vi "manage loss communication.vi"(8 "error in (no error)":errorcluster, 11 "Channel in":refnum<class "Channel.lvclass">) -> (0 "error out":errorcluster, 3 "Channel out":refnum<class "Channel.lvclass">)   [LabVIEW 2018, in "Channel.lvclass"]
uses:
  Channel.lvclass
  Server/Server.lvclass
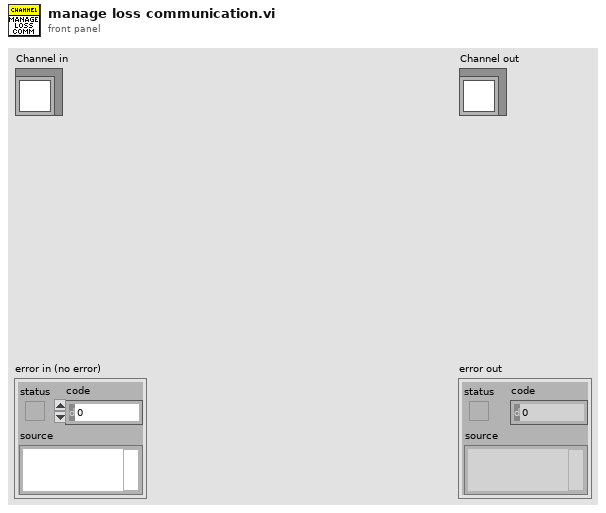
[diagram p1: front panel]
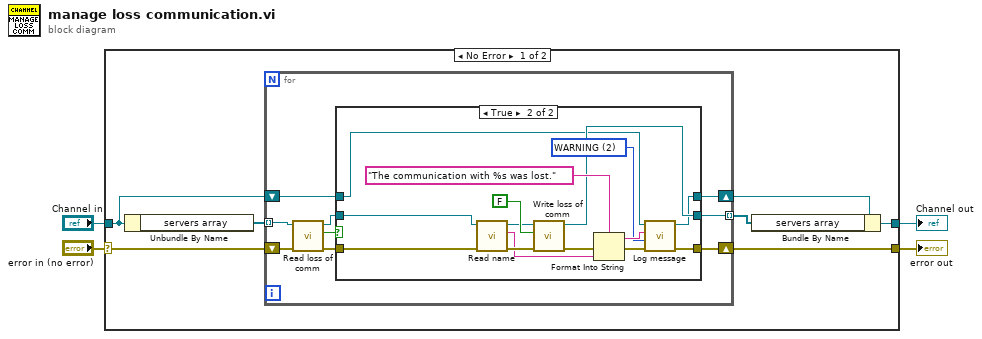
[diagram p0: block diagram]
diagram:
  n1 = case shown="No Error" "error in (no error)" {
    selector: "error in (no error)" -> [w10 w40]
    tunnel: [w9 w40] -> w3
    tunnel: [w7 w39] -> w1
    tunnel: "Channel in" -> [w11 w39]
    frame No Error {
      n2 = Unbundle By Name(w11) -> ("servers array"=w6:refnum<class "Server.lvclass">[])
      n3 = for {
        shift-right: [w19] -> w8
        shift-left: w11 -> [w20]
        shift-right: [w18] -> w9
        shift-left: w10 -> [w15]
        tunnel: w6 -> [w16] mode=indexing
        tunnel: [w12] -> w5 mode=indexing
        n4 = call-dynamic "Read loss of comm.vi"("error in (no error)"=w15, "Server in"=w16) -> ("error out"=w14:errorcluster, "loss of comm"=w13:bool, "Server out"=w17:refnum<class "Server.lvclass">)  [unwired: 7 in]
        n5 = case shown="True" w13 {
          tunnel: w20 -> [w23 w26]
          tunnel: [w23 w25] -> w19
          tunnel: [w22 w27] -> w18
          tunnel: w17 -> [w21 w34]
          tunnel: w14 -> [w22 w33]
          tunnel: [w21 w35] -> w12
          frame False {
          }
          frame True {
            w24 = u16 2 items=[" DEBBUG ", "  INFO  ", "WARNING ", " ERROR  ", "CRITICAL"] ("log level")
            n6 = call-dynamic "Read name.vi"("error in (no error)"=w33, "Server in"=w34) -> ("error out"=w32:errorcluster, "name"=w30:string, "Server out"=w31:refnum<class "Server.lvclass">)  [unwired: 7 in]
            n7 = call-dynamic "Write loss of comm.vi"("error in (no error)"=w32, "loss of comm"=FALSE, "Server in"=w31) -> ("error out"=w37:errorcluster, "Server out"=w35:refnum<class "Server.lvclass">)  [unwired: 7 in]
            n8 = Format Into String(format string="The communication with %s was lost.", error in=w37, w30) -> (resulting string=w29:string, error out=w28:errorcluster)  [unwired: 1 in]
            n9 = call "Log message.vi"("error in (no error)"=w28, "log level"=w24, "String"=w29, "Channel in"=w26) -> ("error out"=w27:errorcluster, "Channel out"=w25:refnum<class "Channel.lvclass">)  [unwired: 6 in]
          }
        }
      }
      n10 = Bundle By Name(cluster=w8, "servers array"=w5) -> (w7:refnum<class "Channel.lvclass">)
    }
    frame Error {
    }
  }
  "error out" <- w3
  "Channel out" <- w1
